vi "Auton Drive Gyro & Encoder Turn Slow.vi"(8 "Angle Setpoint":dbl=90.0, 10 "Distance Set Point":dbl) -> (3 "At Destination?":bool=TRUE)   [LabVIEW 2014]
uses:
  <vilib>/Rock Robotics/WPI/RobotDrive/WPI_RobotDriveGetSetRefNum.vi
  <vilib>/addons/control/pid/pid.llb/PID (DBL).vi
  <vilib>/Rock Robotics/Network Tables/SD Write Number.vi
  <vilib>/Rock Robotics/WPI/RobotDrive/WPI_RobotDriveArcadeDrive_ButtonSpin.vi
  <vilib>/addons/control/pid/NI_PID_pid.lvlib
panel:
  in  "Dead Zone":dbl=0.4
  out "In range gyro?":bool=TRUE
  in  "Gyro Destination Range":dbl=1.5
  out "Y Value Forward/Rev":dbl=0.5815437067645106 format="%.2f"
  in  "Gyro Gains":T1={"proportional gain (Kc)"=0.35, "integral time (Ti, min)"=0.0, "derivative time (Td, min)"=0.0} {"derivative time (Td, min)" format="%.3f"; "integral time (Ti, min)" format="%.3f"; "proportional gain (Kc)" format="%.3f"}
  in  "Gyro Range":cluster{"output high":dbl, "output low":dbl}={"output high"=0.7, "output low"=-0.7} {"output low" format="%.2f"; "output high" format="%.2f"}
  out "Gyro Reading":dbl(knob)=88.17958155398 scale=-180.0..180.0
  in  "Gain (VoltsPerDegree/Second)":dbl=0.0066
  in  "Gains":T1={"proportional gain (Kc)"=0.1666, "integral time (Ti, min)"=0.0, "derivative time (Td, min)"=0.0} {"derivative time (Td, min)" format="%.3f"; "integral time (Ti, min)" format="%.3f"; "proportional gain (Kc)" format="%.3f"}
  in  "Range":cluster{"output high":dbl, "output low":dbl}={"output high"=0.7, "output low"=-0.7} {"output low" format="%.2f"; "output high" format="%.2f"}
  # "Robot Room Floor\nHigh .5\nLow -.5\nDead Zone .1\nProportional gain .033"
  # "Field surface\nHigh .8\nLow -.8 \nDead Zone .4\nProportional gain .033"
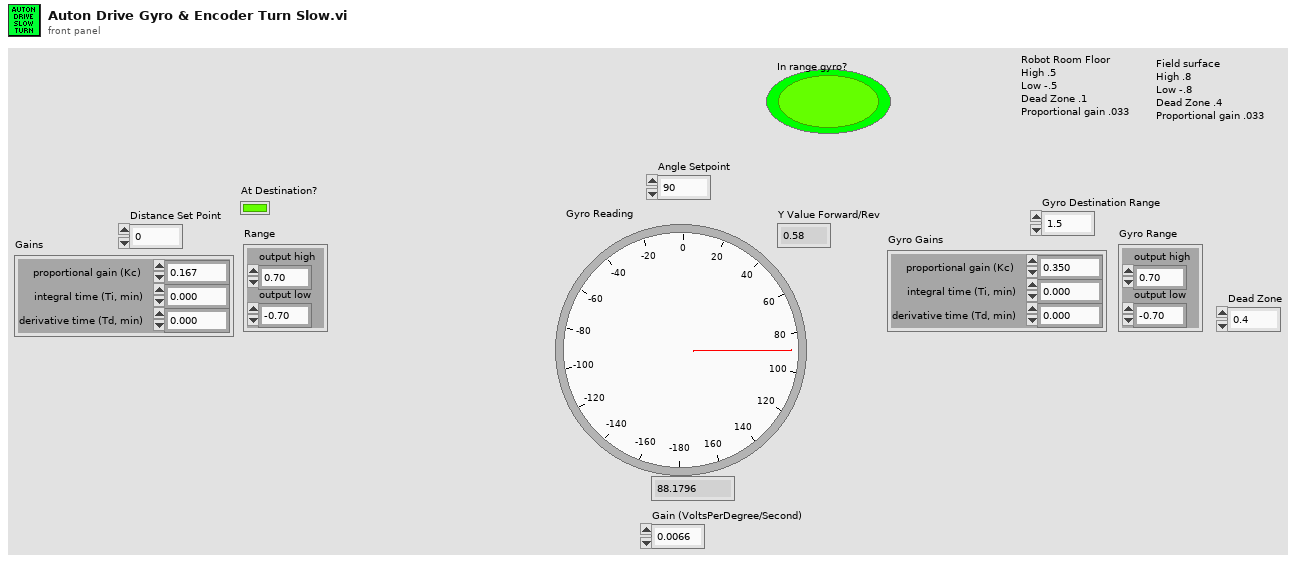
[diagram p1: front panel]
types:
  T1 = cluster{"proportional gain (Kc)":dbl, "integral time (Ti, min)":dbl, "derivative time (Td, min)":dbl}
  T2 = typedef "WPI_GyroDevRef.ctl" = cluster{"DevStatus":errorcluster, "Analog Module":T3, "Analog Channel":T4, "Offset":dbl, "Gain (VoltsPerDegree/Second)":dbl}
  T3 = typedef "FPGA_TypedefAnalogModule.ctl" = enum16{"Controller 1"}
  T4 = typedef "FPGA_AIChannel.ctl" = enum8{"AI 0", "AI 1", "AI 2", "AI 3", "AI MXP 0", "AI MXP 1", "AI MXP 2", "AI MXP 3", "Invalid"}
  T5 = typedef "WPI_EncoderDevRef.ctl" = cluster{"DevStatus":errorcluster, "EncoderIndex":T6, "CounterIndex":T7, "DistancePerCount":dbl, "Decoding Type":T8}
  T6 = typedef "FPGA_EncoderIdx.ctl" = enum8{"Enc 0", "Enc 1", "Enc 2", "Enc 3", "Enc 4", "Enc 5", "Enc 6", "Enc 7", "Invalid"}
  T7 = typedef "FPGA_CounterCtrSystemIndex.ctl" = enum8{"Ctr 0", "Ctr 1", "Ctr 2", "Ctr 3", "Ctr 4", "Ctr 5", "Ctr 6", "Ctr 7", "Invalid"}
  T8 = typedef "WPI_EncoderType.ctl" = enum16{"1x", "2x", "4x"}
  T9 = typedef "WPI_RobotDriveDevRef.ctl" = cluster{"DevStatus":errorcluster, "Motors[]":T10[], "Square Inputs":bool, "Max Output":dbl}
  T10 = typedef "WPI_MotorControlDeviceRef.ctl" = cluster{"DeviceStatus":errorcluster, "Type":T11, "PWM":cluster{"Controller":T12, "PWM Channel":T13, "DeadBand":T14}, "CAN":cluster{"Device Number":u8, "Control Mode":T15, "Semaphore":T16, "Max Vout":dbl, "TalonSRX Control Mode":T17}, "Invert":bool, "TransformRef":T18, "InvTransformRef":T18}
  T11 = typedef "WPI_MotorControlType.ctl" = enum16{"PWM", "CAN", "CANTalonSRX"}
  T12 = typedef "FPGA_TypedefDigitalModule.ctl" = enum16{"Controller 1"}
  T13 = typedef "FPGA_DIOPWMChannel.ctl" = enum8{"PWM 0", "PWM 1", "PWM 2", "PWM 3", "PWM 4", "PWM 5", "PWM 6", "PWM 7", "PWM 8", "PWM 9", "PWM MXP 0", "PWM MXP 1", "PWM MXP 2", "PWM MXP 3", "PWM MXP 4", "PWM MXP 5", "PWM MXP 6", "PWM MXP 7", "PWM MXP 8", "PWM MXP 9", "Invalid"}
  T14 = typedef "WPI_PWMDeadband.ctl" = cluster{"Name":string, "maxPositivePwm":i32, "minPositivePwm":i32, "centerPwm":i32, "maxNegativePwm":i32, "minNegativePwm":i32, "angularRange":u16}
  T15 = typedef "WPI_CANJaguar_ControlMode.ctl" = enum8{"Percent VBus", "Current", "Speed", "Position", "Voltage"}
  T16 = typedef "Semaphore RefNum" = refnum<k1>
  T17 = typedef "WPI_CANTalonSRX_APIControlMode.ctl" = enum8{"Percent VBus", "Speed", "Position", "Slave", "Unchanged / Invalid"}
  T18 = typedef "WPI_PWMTransform_ConPane.ctl" = refnum<vi>
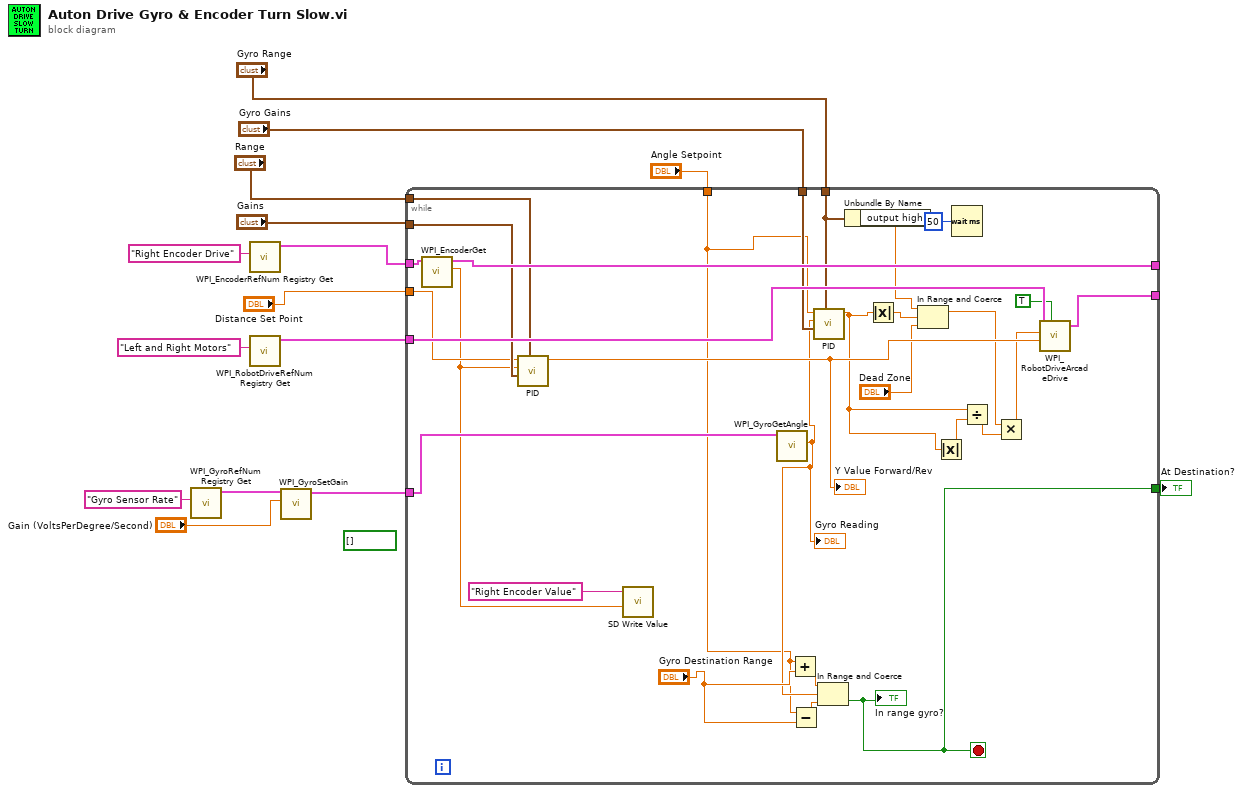
[diagram p0: block diagram]
diagram:
  (unwired) bool[] []
  n1 = call <vilib>:"WPI_GyroRefNum Registry Get.vi"("refnum name"="Gyro Sensor Rate") -> ("GyroDevRef"=w8:T2)  [unwired: 9 in, 1 out]
  n2 = call <vilib>:"WPI_EncoderRefNum Registry Get.vi"("refnum name"="Right Encoder Drive") -> ("EncoderDevRef"=w12:T5)  [unwired: 9 in, 1 out]
  n3 = call <vilib>:"WPI_RobotDriveRefNum Registry Get.vi"("refnum name"="Left and Right Motors") -> ("RobotDriveDevRef"=w14:T9)  [unwired: 9 in, 1 out]
  n4 = call <vilib>:"WPI_GyroSetGain.vi"("Gain (VoltsPerDegree/Second)"="Gain (VoltsPerDegree/Second)", "GyroDevRef"=w8) -> ("GyroDevRef"=w7:T2)  [unwired: 1 in, 8 out]
  n5 = while {
    tunnel: [w43] -> _
    tunnel: [w39] -> _
    tunnel: w14 -> [w38]
    tunnel: w12 -> [w42]
    tunnel: "Distance Set Point" -> [w34]
    tunnel: w7 -> [w40]
    tunnel: "Range" -> [w36]
    tunnel: "Gains" -> [w35]
    tunnel: "Gyro Range" -> [w17]
    tunnel: "Gyro Gains" -> [w37]
    tunnel: "Angle Setpoint" -> [w27]
    tunnel: [w26] -> w1
    stop <- w26 stop-if-true
    n6 = call <vilib>:"WPI_EncoderGet.vi"("EncoderDevRef"=w42) -> ("Distance"=w33:dbl, "EncoderDevRef"=w43:T5)  [unwired: 5 in, 4 out]
    n7 = call-poly <vilib>:"PID.vi"("output range"=w36, "PID gains"=w35, "process variable"=w33, "setpoint"=w34) -> ("output"=w32:dbl)  [unwired: 6 in, 1 out]
    "Y Value Forward/Rev" <- w32
    n8 = call-poly <vilib>:"SD Write Value.vi"("Numeric"=w33, "Name"="Right Encoder Value") -> ()  [unwired: 8 in, 2 out]
    n9 = call <vilib>:"WPI_GyroGetAngle.vi"("GyroDevRef"=w40) -> ("Angle"=w28:dbl)  [unwired: 1 in, 9 out]
    "Gyro Reading" <- w28
    n10 = Add(x=w27, y="Gyro Destination Range") -> (x+y=w30:dbl)
    n11 = Subtract(x=w27, y="Gyro Destination Range") -> (x-y=w31:dbl)
    n12 = call-poly <vilib>:"PID.vi"("output range"=w17, "PID gains"=w37, "process variable"=w28, "setpoint"=w27) -> ("output"=w19:dbl)  [unwired: 6 in, 1 out]
    n13 = In Range and Coerce(upper limit=w30, x=w28, lower limit=w31) -> (In Range?=w26:bool)  [unwired: 1 out]
    "In range gyro?" <- w26
    n14 = Unbundle By Name(w17) -> ("output high"=w16:dbl)
    n15 = Absolute Value(x=w19) -> (abs(x)=w18:dbl)
    n16 = In Range and Coerce(upper limit=w16, x=w18, lower limit="Dead Zone") -> (coerced(x)=w22:dbl)  [unwired: 1 out]
    n17 = Absolute Value(x=w19) -> (abs(x)=w23:dbl)
    n18 = Wait (ms)(milliseconds to wait=u32 50) -> ()  [unwired: 1 out]
    n19 = Divide(x=w19, y=w23) -> (x/y=w21:dbl)
    n20 = Multiply(x=w22, y=w21) -> (x*y=w20:dbl)
    n21 = call-poly <vilib>:"WPI_RobotDriveArcadeDrive.vi"("Spin?"=TRUE, "Y axis value"=w32, "X axis value"=w20, "RobotDriveDevRef"=w38) -> ("RobotDriveDevRef"=w39:T9)  [unwired: 5 in, 2 out]
  }
  "At Destination?" <- w1
